vi "2 check_inside_square.vi"(9 "UTM Location":T1 {"North" format="%#_10f"; "East" format="%#_8f"}, 10 "StationKeeping.lvclass":refnum<class "StationKeeping.lvclass">) -> (2 "In Square?":bool)   [LabVIEW 2011]
doc: "To check if the boat is inside the StationKeeping square, 4 triangle areas are calculated. Each pair of adjacent station corners are used with the boat's position. If the boat is in the station, this will equal the area of the station. If the boat is outside the station, it will be larger. The -10 constant is a buffer, in case of any error, so the timer definitely starts."
uses:
  2 Typedefs/UTM Location.ctl
  2 Classes/Missions/StationKeeping/StationKeeping.lvclass
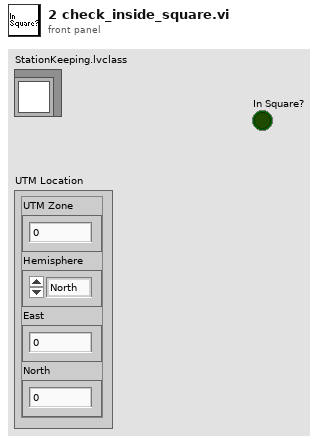
[diagram p1: front panel]
types:
  T1 = typedef "UTM Location.ctl" = cluster{"UTM Zone":dbl, "Hemisphere":enum16{"North", "South"}, "East":dbl, "North":dbl}
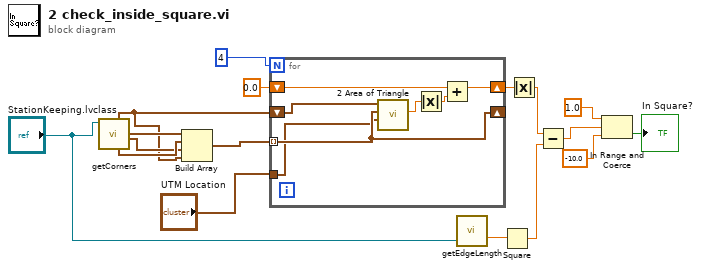
[diagram p0: block diagram]
diagram:
  n1 = call-dynamic "getCorners.vi"("StationKeeping in"="StationKeeping.lvclass") -> ("Buoy SW"=w16:T1, "Buoy NE"=w12:T1, "Buoy SE"=w17:T1, "Buoy NW"=w11:T1)  [unwired: 5 in, 2 out]
  n2 = Build Array(w12, w17, w16, w11) -> (w15:T1[])
  n3 = for {
    N: 4 -> [_]
    tunnel: w15 -> [w23] mode=indexing
    tunnel: "UTM Location" -> [w22]
    shift-right: [w23] -> _
    shift-left: w11 -> [w24]
    shift-right: [w20] -> w7
    shift-left: 0.0 -> [w19]
    n4 = call "2 Area of Triangle.vi"("pt C"=w22, "pt B"=w23, "pt A"=w24) -> ("Area"=w21:dbl)  [unwired: 8 in]
    n5 = Absolute Value(x=w21) -> (abs(x)=w18:dbl)
    n6 = Add(x=w19, y=w18) -> (x+y=w20:dbl)
  }
  n7 = call "getEdgeLength.vi"("StationKeeping in"="StationKeeping.lvclass") -> ("Edge Length"=w8:dbl)  [unwired: 9 in, 1 out]
  n8 = Square(x=w8) -> (x^2=w6:dbl)
  n9 = Absolute Value(x=w7) -> (abs(x)=w1:dbl)
  n10 = Subtract(x=w1, y=w6) -> (x-y=w5:dbl)
  n11 = In Range and Coerce(upper limit=1.0, x=w5, lower limit=-10.0) -> (In Range?=→"In Square?":bool)  [unwired: 1 out]
